vi "SetParam.vi"(8 "error in (no error)":errorcluster caption="entrée d'erreur (pas d'erreur)", 10 "FeatureHasher":T1={"n_features"=1048576, "input_type"="dict", "dtype"="float", "alternate_sign"=TRUE}, 11 "FeatureHasher.lvclass":refnum<class "FeatureHasher.lvclass">) -> (0 "error out":errorcluster caption="sortie d'erreur", 3 "FeatureHasher.lvclass":refnum<class "FeatureHasher.lvclass">)   [LabVIEW 2020, in "FeatureHasher.lvclass"]
doc: "Set Parameters"
uses:
  FeatureHasher.lvclass
  FeatureHasher.lvclass/FeatureHasher.ctl
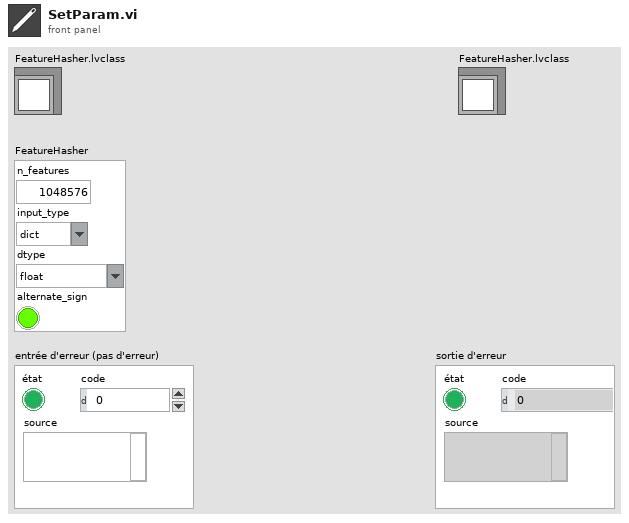
[diagram p1: front panel]
types:
  T1 = cluster{"n_features":i32, "input_type":string, "dtype":string, "alternate_sign":bool}
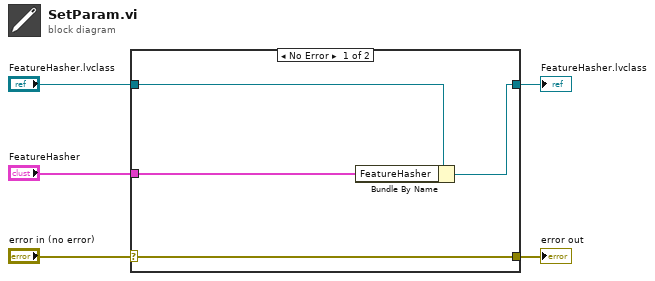
[diagram p0: block diagram]
diagram:
  n1 = case shown="No Error" "error in (no error)" {
    selector: "error in (no error)" -> [w9 w10]
    tunnel: [w9 w10] -> w4
    tunnel: [w7 w11] -> w2
    tunnel: "FeatureHasher.lvclass" -> [w8 w11]
    tunnel: "FeatureHasher" -> [w6 _]
    frame No Error {
      n2 = Bundle By Name(cluster=w8, "FeatureHasher"=w6) -> (w7:refnum<class "FeatureHasher.lvclass">)
    }
    frame Error {
    }
  }
  "error out" <- w4
  "FeatureHasher.lvclass" <- w2
